vi "Cargo Intake.vi"   [LabVIEW 2018]
uses:
  <vilib>/Rock Robotics/WPI/Solenoid/WPI_SolenoidChannel.ctl
  <vilib>/Rock Robotics/SystemInterfaces/DIO/FPGA_DIOChannel.ctl
  <vilib>/Rock Robotics/WPI/ThirdParty/Phoenix-LabVIEW/Motor Controller/Controls/CTRE_Phoenix_MotorControl_ControlMode.ctl
  <vilib>/Rock Robotics/WPI/Solenoid/WPI_SolenoidValue.ctl
  Cargo Intake Global.vi
  <vilib>/Rock Robotics/WPI/Solenoid/WPI_SolenoidOpenSingle.vi
  Sensors/Sensors Global.vi
  Times/Times Global.vi
  <vilib>/Rock Robotics/WPI/Solenoid/WPI_SolenoidSetEnum.vi
types:
  T1 = typedef "FPGA_DIOChannel.ctl" = enum8{"DIO 0", "DIO 1", "DIO 2", "DIO 3", "DIO 4", "DIO 5", "DIO 6", "DIO 7", "DIO 8", "DIO 9", "DIO MXP 0", "DIO MXP 1", "DIO MXP 2", "DIO MXP 3", "DIO MXP 4", "DIO MXP 5", "DIO MXP 6", "DIO MXP 7", "DIO MXP 8", "DIO MXP 9", "DIO MXP 10", "DIO MXP 11", "DIO MXP 12", "DIO MXP 13", "DIO MXP 14", "DIO MXP 15", "SPI Port CS1", "SPI Port CS2", "SPI Port CS3", "SPI Port MISO", "SPI Port MOSI", "Invalid"}
  T2 = typedef "WPI_SolenoidChannel.ctl" = enum8{"Solenoid 0", "Solenoid 1", "Solenoid 2", "Solenoid 3", "Solenoid 4", "Solenoid 5", "Solenoid 6", "Solenoid 7", "Invalid"}
  T3 = enum16{"Full Manual Control", "Manual Control", "Automated Control"}
  T4 = typedef "WPI_SolenoidValue.ctl" = enum16{"Off", "On", "Forward", "Reverse"}
  T5 = typedef "WPI_SolenoidDevRef.ctl" = cluster{"DevStatus":errorcluster, "Pneumatics Control Module":u8, "Forward Solenoid Channel":T2, "Reverse Solenoid Channel":T2}
  T6 = typedef "WPI_DigitalInputDevRef.ctl" = cluster{"DevStatus":errorcluster, "DIO Channel":T1}
  T7 = typedef "WPI_MotorControlDeviceRef.ctl" = cluster{"DeviceStatus":errorcluster, "Type":T8, "PWM":cluster{"PWM Channel":T9, "DeadBand":T10}, "CAN":cluster{"Device Number":u8, "SetOutput VI Ref":variant, "GetOutput VI Ref":variant, "Enable VI Ref":variant, "Disable VI Ref":variant, "Data":variant}, "Invert":bool, "DIO PWM":cluster{"PWM \"Enable\" Channel":T9, "DIOChannel":T1, "PWM Rate":dbl}}
  T8 = typedef "WPI_MotorControlType.ctl" = enum16{"PWM", "CAN", "DIO PWM"}
  T9 = typedef "FPGA_DIOPWMChannel.ctl" = enum8{"PWM 0", "PWM 1", "PWM 2", "PWM 3", "PWM 4", "PWM 5", "PWM 6", "PWM 7", "PWM 8", "PWM 9", "PWM MXP 0", "PWM MXP 1", "PWM MXP 2", "PWM MXP 3", "PWM MXP 4", "PWM MXP 5", "PWM MXP 6", "PWM MXP 7", "PWM MXP 8", "PWM MXP 9", "Invalid"}
  T10 = typedef "WPI_PWMDeadband.ctl" = cluster{"Name":string, "maxPositivePwm":i32, "minPositivePwm":i32, "centerPwm":i32, "maxNegativePwm":i32, "minNegativePwm":i32, "angularRange":u16}
  T11 = typedef "CTRE_Phoenix_MotorControl_ControlMode.ctl" = u16
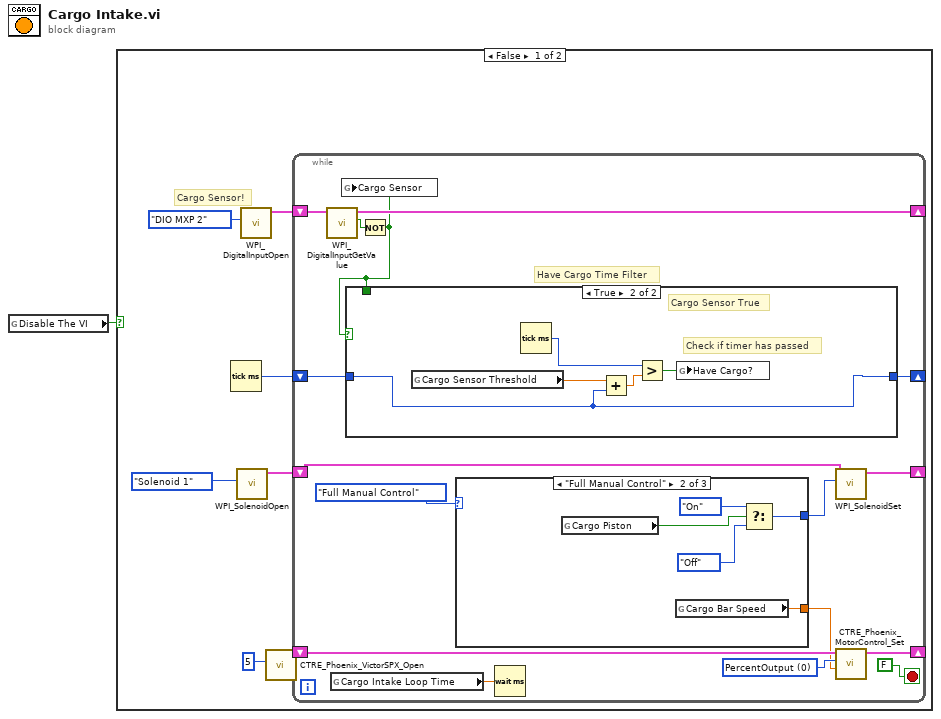
[diagram p0: block diagram]
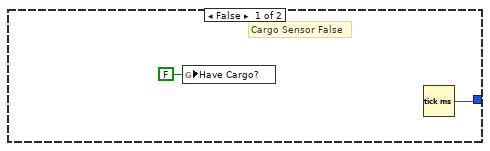
[diagram p2: hidden frame]
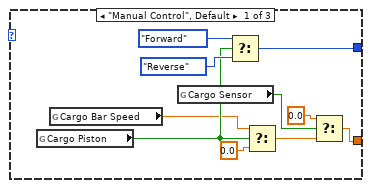
[diagram p3: hidden frame]
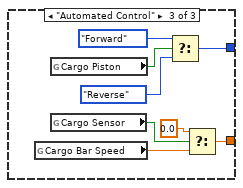
[diagram p4: hidden frame]
diagram:
  n1 = global read "Cargo Intake Global.vi" "Disable The VI"() -> (w1:bool)
  n2 = case shown="False" w1 {
    frame False {
      # "Cargo Sensor!"
      n3 = Tick Count (ms)() -> (millisecond timer value=w2:u32)
      n4 = call-poly <vilib>:"WPI_SolenoidOpen.vi"("Solenoid Channel"=WPI_SolenoidChannel."Solenoid 1") -> ("SolenoidDevRef"=w5:T5)  [unwired: 9 in, 1 out]
      n5 = call <vilib>:"WPI_DigitalInputOpen.vi"("DIO Channel"=FPGA_DIOChannel."DIO MXP 2") -> ("DigitalInputDevRef"=w4:T6)  [unwired: 9 in, 1 out]
      n6 = call <vilib>:"CTRE_Phoenix_VictorSPX_Open.vi"("Device Number"=u8 5) -> ("CAN Talon SRX Ref"=w7:T7)  [unwired: 9 in, 1 out]
      n7 = while {
        shift-right: [w21] -> _
        shift-left: w7 -> [w19]
        shift-right: [w17] -> _
        shift-left: w5 -> [w15]
        shift-right: [w13] -> _
        shift-left: w4 -> [w14]
        shift-right: [w11] -> _
        shift-left: w2 -> [w12]
        stop <- FALSE stop-if-true
        w20 = T11 0 items=["PercentOutput"=0, "Position"=1, "Velocity"=2, "Current"=3, "Follower"=5, "MotionProfile"=6, "MotionMagic"=7, "MotionProfileArc"=10, "Disabled"=15] ("Control Mode")
        # "Have Cargo Time Filter"
        n8 = call <vilib>:"WPI_DigitalInputGetValue.vi"("DigitalInputDevRef"=w14) -> ("Value"=w10:bool, "DigitalInputDevRef"=w13:T6)  [unwired: 8 in, 1 out]
        n9 = global read "Times Global.vi" "Cargo Intake Loop Time"() -> (w24:dbl)
        n10 = Not(x=w10) -> (.not. x?=w9:bool)
        n11 = global write "Cargo Intake Global.vi" "Cargo Sensor"(w9) -> ()
        n12 = case shown="True" w9 {
          tunnel: w12 -> [_ w28]
          tunnel: [w25 w28] -> w11
          tunnel: w9 -> [_ _]
          frame False {
            # "Cargo Sensor False"
            n13 = global write "Cargo Intake Global.vi" "Have Cargo?"(FALSE ("Have Cargo?")) -> ()
            n14 = Tick Count (ms)() -> (millisecond timer value=w25:u32)
          }
          frame True {
            # "Check if timer has passed"
            # "Cargo Sensor True"
            n15 = global read "Cargo Intake Global.vi" "Cargo Sensor Threshold"() -> (w27:dbl)
            n16 = Tick Count (ms)() -> (millisecond timer value=w30:u32)
            n17 = Add(x=w27, y=w28) -> (x+y=w29:dbl)
            n18 = Greater?(x=w30, y=w29) -> (0:w31:bool)
            n19 = global write "Cargo Intake Global.vi" "Have Cargo?"(w31) -> ()
          }
        }
        n20 = case shown="\"Full Manual Control\"" T3."Full Manual Control" ("Cargo Intake Mode") {
          tunnel: [w39 w46 w54] -> w18
          tunnel: [w35 w43 w49] -> w16
          frame "Manual Control", Default {
            n21 = global read "Cargo Intake Global.vi" "Cargo Piston"() -> (w33:bool)
            n22 = global read "Cargo Intake Global.vi" "Cargo Bar Speed"() -> (w32:dbl)
            n23 = global read "Sensors Global.vi" "Cargo Sensor"() -> (w34:bool)
            n24 = Select(t=WPI_SolenoidValue."Forward" ("Value"), s=w33, f=WPI_SolenoidValue."Reverse" ("Value")) -> (s? t:f=w35:T4)
            n25 = Select(t=w32, s=w33, f=0.0 ("t")) -> (s? t:f=w41:dbl)
            n26 = Select(t=0.0, s=w34, f=w41) -> (s? t:f=w39:dbl)
          }
          frame "Full Manual Control" {
            n27 = global read "Cargo Intake Global.vi" "Cargo Piston"() -> (w42:bool)
            n28 = global read "Cargo Intake Global.vi" "Cargo Bar Speed"() -> (w46:dbl)
            n29 = Select(t=WPI_SolenoidValue."On" ("Value"), s=w42, f=WPI_SolenoidValue."Off" ("Value")) -> (s? t:f=w43:T4)
          }
          frame "Automated Control" {
            n30 = global read "Cargo Intake Global.vi" "Cargo Bar Speed"() -> (w52:dbl)
            n31 = global read "Cargo Intake Global.vi" "Cargo Piston"() -> (w48:bool)
            n32 = global read "Sensors Global.vi" "Cargo Sensor"() -> (w47:bool)
            n33 = Select(t=WPI_SolenoidValue."Forward" ("Value"), s=w48, f=WPI_SolenoidValue."Reverse" ("Value")) -> (s? t:f=w49:T4)
            n34 = Select(t=0.0, s=w47, f=w52) -> (s? t:f=w54:dbl)
          }
        }
        n35 = Wait (ms)(milliseconds to wait=w24) -> ()  [unwired: 1 out]
        n36 = call-poly <vilib>:"WPI_SolenoidSet.vi"("Value"=w16, "SolenoidDevRef"=w15) -> ("SolenoidDevRef"=w17:T5)  [unwired: 8 in, 1 out]
        n37 = call <vilib>:"CTRE_Phoenix_MotorControl_Set.vi"("Output"=w18, "Control Mode"=w20, "PhoenixMotorControlDevRef"=w19) -> ("PhoenixMotorControlDevRef"=w21:T7)  [unwired: 7 in, 1 out]
      }
    }
    frame True {
    }
  }
